vi "Compute_Implied_Links.vi"(8 "Check front panel exclusion?":bool, 9 "File":T2, 10 "Linker:Read Info From File":T3(array[cluster]), 11 "AB_Source.lvclass":refnum<class "AB_Source.lvclass">) -> (0 "Exclude front panel? (false if not checking)":bool, 1 "links":u32[](array[numeric]))   [LabVIEW 2020, in "AB_Source.lvclass"]
uses:
  <vilib>/AppBuilder/AB_Classes/Source/AB_Source.lvclass
  <vilib>/Utility/lvfile.llb/LVFileType.ctl
  <vilib>/AppBuilder/AB_Source_Property_Type.ctl
  <vilib>/Utility/lvfile.llb/NI_FileType.lvlib
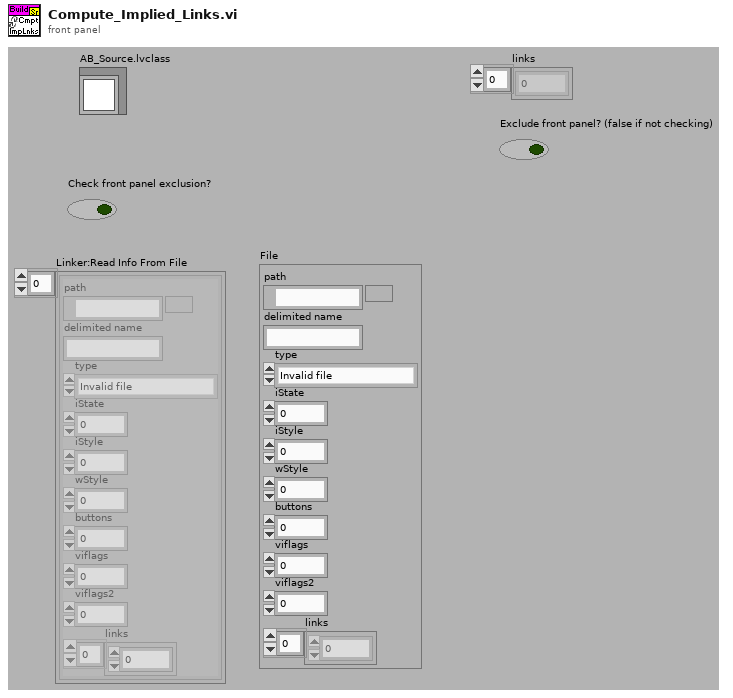
[diagram p1: front panel]
types:
  T1 = typedef "NI_FileType.lvlib/LVFileType.ctl" = enum32{"Invalid file", "Unknown type", "Instrument", "Control", "Polymorphic VI", "Project", "Library", "LVClass", "XControl", "XNode", "Shared library", ".NET assembly", "ActiveX interface", "CIN", "Run-time menu", "Palette menu", "Help file", "LLB", "XNode Edit Dependency", "Class Private Data Control", "Statechart", "MathScript .m file", "Ladder Diagram", "LVLibp", "XNode Build Dependency"}
  T2 = cluster{"path":path, "delimited name":string, "type":T1, "iState":u32, "iStyle":u16, "wStyle":u16, "buttons":u16, "viflags":u32, "viflags2":u32, "links":u32[]}
  T3 = cluster{"path":path, "delimited name":string, "type":T1, "iState":u32, "iStyle":u16, "wStyle":u16, "buttons":u16, "viflags":u32, "viflags2":u32, "links":u32[]}[]
  T4 = typedef "AB_Source_Property_Type.ctl" = enum16{"Remove block diagram", "Remove front panel", "Password", "Window has title bar", "Show menu bar", "Show vertical scroll bar", "Show horizontal scroll bar", "Show toolbar", "Show Abort button", "Show fp when called", "Window behavior", "Allow user to close window", "Window run-time position", "Run when opened", "Allow debugging", "Auto error handling", "Generate guard code", "Use stack variables", "Expression folding", "Integer only", "Inline subVI"}
  T5 = typedef "AB_Source_Properties.ctl" = cluster{"sourcePropertyType":T4, "value":variant}
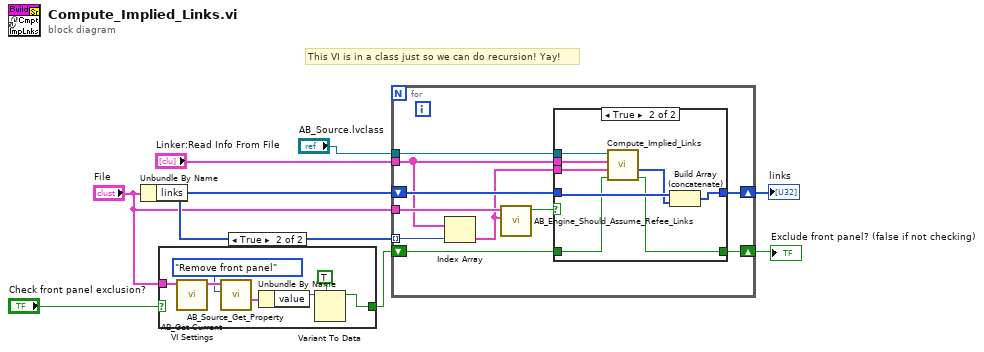
[diagram p0: block diagram]
diagram:
  # "This VI is in a class just so we can do recursion! Yay!"
  n1 = Unbundle By Name("File") -> ("links"=w8:u32[])
  n2 = case shown="True" "Check front panel exclusion?" {
    selector: "Check front panel exclusion?" -> [w9 _]
    tunnel: "File" -> [_ w11]
    tunnel: [w9 w10] -> w1
    frame False {
    }
    frame True {
      n3 = call <vilib>:"AB_Get Current VI Settings.vi"("linkerInfo"=w11) -> ("sourceProperties"=w13:T5[])  [unwired: 10 in]
      n4 = call <vilib>:"AB_Source_Get_Property.vi"("type"=AB_Source_Property_Type."Remove front panel", "sourceProperties in"=w13) -> ("sourceProperty"=w16:T5)  [unwired: 6 in, 3 out]
      n5 = Unbundle By Name(w16) -> ("value"=w14:variant)
      n6 = Variant To Data(type=TRUE, Variant=w14) -> (data=w10:bool)  [unwired: 1 in, 1 out]
    }
  }
  n7 = for {
    tunnel: w8 -> [w21] mode=indexing
    shift-right: [w19] -> w5
    shift-left: w8 -> [w24]
    tunnel: "File" -> [w26]
    tunnel: "AB_Source.lvclass" -> [w23]
    shift-right: [w17] -> w4
    shift-left: w1 -> [w18]
    tunnel: "Linker:Read Info From File" -> [w22]
    n8 = Index Array(array=w22, index=w21) -> (element=w20:T2)
    n9 = call <vilib>:"AB_Engine_Should_Assume_Refee_Links.vi"("Refee"=w20, "Refer"=w26) -> ("Assume refee links?"=w25:bool)  [unwired: 9 in]
    n10 = case shown="True" w25 {
      tunnel: w24 -> [w28 w34]
      tunnel: w23 -> [_ w36]
      tunnel: w22 -> [_ w35]
      tunnel: w20 -> [_ w32]
      tunnel: [w28 w33] -> w19
      tunnel: w18 -> [w27 w31]
      tunnel: [w27 w30] -> w17
      frame False {
      }
      frame True {
        n11 = call-dynamic "Compute_Implied_Links.vi"("Check front panel exclusion?"=w31, "File"=w32, "Linker:Read Info From File"=w35, "AB_Source.lvclass"=w36) -> ("Exclude front panel? (false if not checking)"=w30:bool, "links"=w29:u32[])  [unwired: 6 in]
        n12 = Build Array (concatenate)(w34, w29) -> (w33:u32[])
      }
    }
  }
  "links" <- w5
  "Exclude front panel? (false if not checking)" <- w4
